vi "Main.vi"() -> ()   [LabVIEW 2019]
uses:
  Typedefs/#enum_MasterState.ctl
  Typedefs/#cluster_GUIRefs.ctl
  SubVIs/Application Configuration VIs/#cluster_AppConfiguration.ctl
  SubVIs/LowLevelError.vi
panel:
  in  "Results Viewer":bool
  in  "POX Data History":string[](array[string])
  in  "Save?":bool caption="Save Results?"
  in  "Measure":bool
  in  "Measurement Directory":path
  in  "Stop":bool
  out "O2 Saturation":dbl(graph)
  out "Heart beat":dbl(graph)
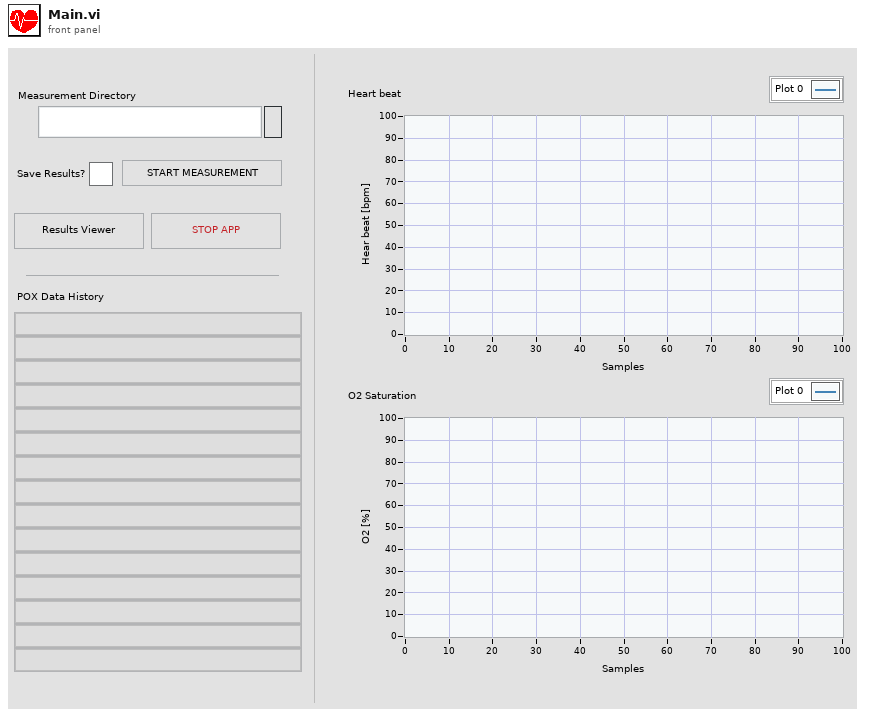
[diagram p1: front panel]
types:
  T1 = typedef "#enum_MasterState.ctl" = enum16{"Idle", "Init", "Close", "Error"}
  T2 = typedef "#cluster_ApplicationData.ctl" = cluster{"Acq Queue":refnum<queue>, "Saving Queue":refnum<queue>}
  T3 = typedef "#cluster_GUIRefs.ctl" = cluster{"Measure":refnum<vi>, "Save?":refnum<vi>, "Stop":refnum<vi>, "Measurement Dir":refnum<vi>, "Heart beat":refnum<vi>, "O2":refnum<vi>, "POX Data History":refnum<vi>}
  T4 = typedef "#cluster_AppConfiguration.ctl" = cluster{"Measurements Directory":path}
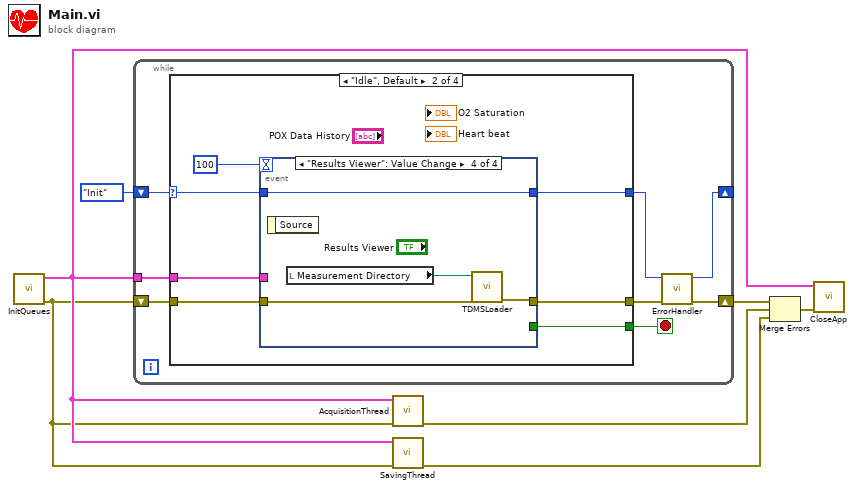
[diagram p0: block diagram]
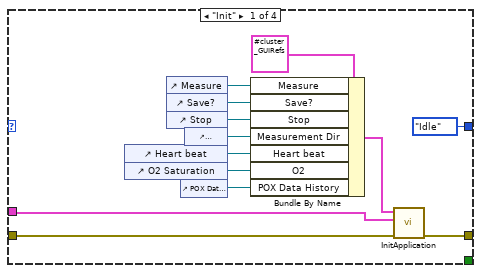
[diagram p2: hidden frame]
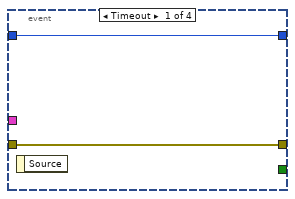
[diagram p3: hidden frame]
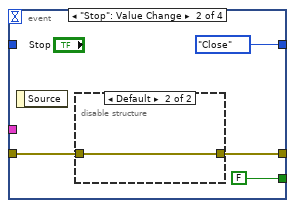
[diagram p4: hidden frame]
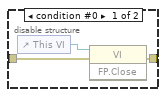
[diagram p5: hidden frame]
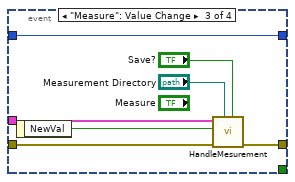
[diagram p6: hidden frame]
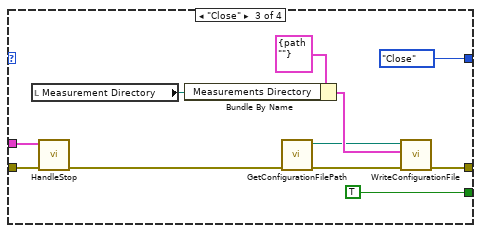
[diagram p7: hidden frame]
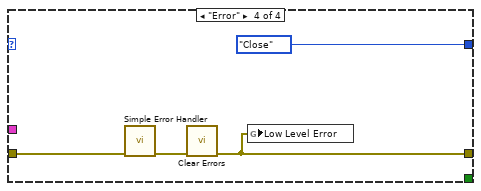
[diagram p8: hidden frame]
diagram:
  n1 = call "InitQueues.vi"() -> ("error out"=w2:errorcluster, "Application Data"=w3:T2)  [unwired: 10 in]
  n2 = while {
    tunnel: w3 -> [w14]
    shift-right: [w10] -> w7
    shift-left: w2 -> [w15]
    shift-right: [w8] -> _
    shift-left: #enum_MasterState."Init" ("Master State") -> [w12]
    stop <- w13 stop-if-true
    n3 = case shown="\"Idle\", Default" w12 {
      selector: w12 -> [_ w31 _ _]
      tunnel: w15 -> [w21 w35 w66 w69]
      tunnel: w14 -> [w18 w34 w63 _]
      tunnel: [w19 w33 w61 w67] -> w11
      tunnel: [_ w32 TRUE _] -> w13
      tunnel: [#enum_MasterState."Idle" ("Master State") w30 #enum_MasterState."Close" ("Master State") #enum_MasterState."Close" ("Master State")] -> w9
      frame "Init" {
        n4 = control-ref of="Heart beat"() -> (w27:refnum<vi>)
        n5 = control-ref of="O2 Saturation"() -> (w28:refnum<vi>)
        n6 = control-ref of="Measure"() -> (w23:refnum<vi>)
        n7 = control-ref of="Save?"() -> (w24:refnum<vi>)
        n8 = control-ref of="Stop"() -> (w25:refnum<vi>)
        n9 = control-ref of="POX Data History"() -> (w16:refnum<vi>)
        n10 = control-ref of="Measurement Directory"() -> (w26:refnum<vi>)
        n11 = Bundle By Name(cluster=T3 {"Measure"=refnum, "Save?"=refnum, "Stop"=refnum, "Measurement Dir"=refnum, "Heart beat"=refnum, "O2"=refnum, "POX Data History"=refnum} ("GUI Refs"), "Measure"=w23, "Save?"=w24, "Stop"=w25, "Measurement Dir"=w26, "Heart beat"=w27, "O2"=w28, "POX Data History"=w16) -> (w20:T3)
        n12 = call "InitApplication.vi"("error in (no error)"=w21, "Application Data in"=w18, "GUI Refs"=w20) -> ("error out"=w19:errorcluster)  [unwired: 8 in]
      }
      frame "Idle", Default {
        n13 = event shown="[3] \"Results Viewer\": Value Change" {
          selector: _ -> [_ _ _ _]
          dyn-events: _ -> [_ _ _ _]
          timeout: 100 -> [_ _ _ _]
          tunnel: w35 -> [w37 w41 w52 w56]
          tunnel: w34 -> [_ _ w50 _]
          tunnel: [w37 w38 w49 w55] -> w33
          tunnel: [_ FALSE _ _] -> w32
          tunnel: w31 -> [w36 _ w46 w53]
          tunnel: [w36 #enum_MasterState."Close" ("Master State") w46 w53] -> w30
          event Timeout {
            n14 = event-data() -> ()  [unwired: 1 in, 1 out]
          }
          event "Stop": Value Change {
            n15 = event-data() -> ()  [unwired: 1 in, 1 out]
            n16 = disable-structure shown="Default" {
              disable-tunnel: w41 -> [w44 w45]
              disable-tunnel: [w43 w45] -> w38
              frame condition #0 {
                n17 = control-ref of="This VI"() -> (w42:refnum<vi>)
                n18 = invoke class="VI" method="FP.Close"(reference=w42, error in=w44) -> (error out=w43:errorcluster)  [unwired: 1 in, 2 out]
              }
              frame condition #1 (active) {
              }
            }
          }
          event "Measure": Value Change {
            n19 = event-data() -> ("NewVal"=w51:bool)  [unwired: 1 in]
            n20 = call "HandleMesurement.vi"("Save?"="Save?", "Measurement Directory"="Measurement Directory", "error in (no error)"=w52, "Measure?"=w51, "Application Data"=w50) -> ("error out"=w49:errorcluster)  [unwired: 6 in]
          }
          event "Results Viewer": Value Change {
            n21 = event-data() -> ()  [unwired: 1 in, 1 out]
            n22 = local read "Measurement Directory"() -> (w54:path)
            n23 = call "TDMSLoader.vi"("Error in"=w56, "Measurements path"=w54) -> ("Error out"=w55:errorcluster)  [unwired: 9 in]
          }
        }
      }
      frame "Close" {
        n24 = local read "Measurement Directory"() -> (w59:path)
        n25 = call "HandleStop.vi"("error in (no error)"=w66, "Application Data"=w63) -> ("error out"=w62:errorcluster)  [unwired: 9 in]
        n26 = Bundle By Name(cluster=T4 {"Measurements Directory"=path ""} ("App Configuration"), "Measurements Directory"=w59) -> (w58:T4)
        n27 = call "GetConfigurationFilePath.vi"() -> ("Configuration File Path"=w57:path)  [unwired: 11 in]
        n28 = call "WriteConfigurationFile.vi"("Error in"=w62, "App Configuration"=w58, "Configuration File Path"=w57) -> ("Error out"=w61:errorcluster)  [unwired: 8 in]
      }
      frame "Error" {
        n29 = call <vilib>:"Simple Error Handler.vi"("error in (no error)"=w69) -> ("error out"=w68:errorcluster)  [unwired: 4 in, 4 out]
        n30 = call <vilib>:"Clear Errors.vi"("error in (no error)"=w68) -> ("error out"=w67:errorcluster)  [unwired: 5 in, 1 out]
        n31 = global write "LowLevelError.vi" "Low Level Error"(w67) -> ()
      }
    }
    n32 = call "ErrorHandler.vi"("error in (no error)"=w11, "Master State in"=w9) -> ("error out"=w10:errorcluster, "Master State out"=w8:T1)  [unwired: 8 in]
  }
  n33 = call "AcquisitionThread.vi"("error in (no error)"=w2, "Application Data"=w3) -> ("error out"=w6:errorcluster)  [unwired: 9 in]
  n34 = call "SavingThread.vi"("error in (no error)"=w2, "Application Data"=w3) -> ("error out"=w1:errorcluster)  [unwired: 9 in]
  n35 = Merge Errors(w7, w6, w1) -> (w5:errorcluster)
  n36 = call "CloseApp.vi"("error in (no error)"=w5, "Application Data"=w3) -> ()  [unwired: 9 in, 1 out]
